vi "Bessel Function Jv.vi"(2 "v":dbl format="%.2f", 3 "x":dbl format="%.2f") -> (1 "Jv(x)":dbl format="%.2f")   [LabVIEW 2020, in "NI_Gmath.lvlib"]
doc: "Computes the Bessel function of the first kind."
uses:
  <vilib>/gmath/NI_Gmath.lvlib
  <resource>/lvanlys.dll
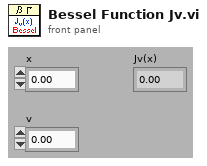
[diagram p1: front panel]
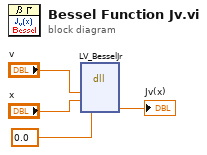
[diagram p0: block diagram]
diagram:
  n1 = dll-call lib="e:/builds/penguin/labview/branches/2020/dev/dist/resource/lvanlys.*" fn="LV_BesselJr"("v"="v", "x"="x", "Jv(x)"=0.0 ("Jr")) -> ("Jv(x)"=→"Jv(x)":dbl)  [unwired: 6 in, 2 out]
